vi "Close serial reference.vi"(8 "error in (no error)":errorcluster, 11 "Serial_comms in":refnum<class "Serial_comms.lvclass">) -> (0 "error out":errorcluster, 3 "Serial_comms out":refnum<class "Serial_comms.lvclass">)   [LabVIEW 2020, in "Serial_comms.lvlib" / "Serial_comms.lvclass"]
uses:
  Serial_comms.lvclass
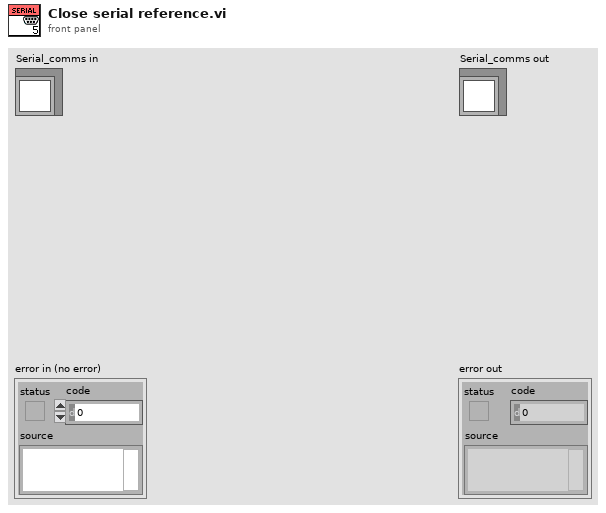
[diagram p1: front panel]
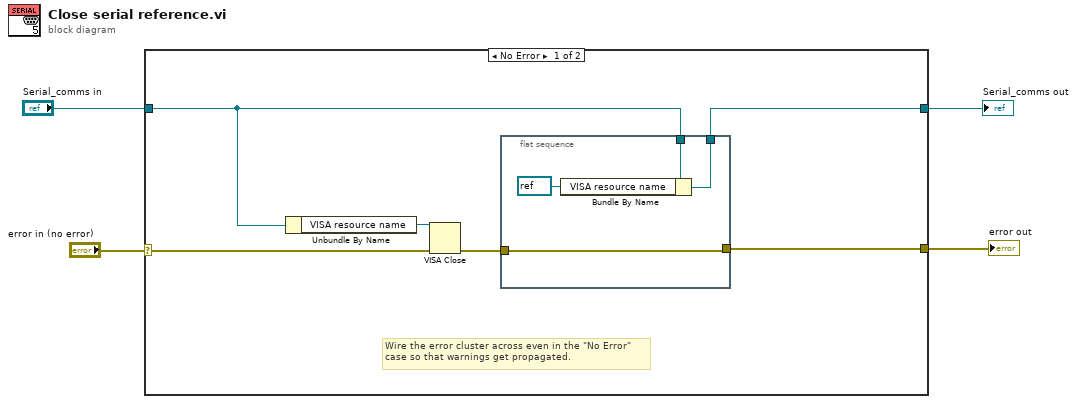
[diagram p0: block diagram]
diagram:
  n1 = case shown="No Error" "error in (no error)" {
    selector: "error in (no error)" -> [w7 w16]
    tunnel: [w6 w16] -> w3
    tunnel: [w5 w15] -> w1
    tunnel: "Serial_comms in" -> [w8 w15]
    frame No Error {
      # "Wire the error cluster across even in the \"No Error\"\ncase so that warnings get propagated."
      n2 = Unbundle By Name(w8) -> ("VISA resource name"=w10:refnum<visa-resource-name>)
      n3 = VISA Close(VISA resource name=w10, error in (no error)=w7) -> (error out=w9:errorcluster)
      n4 = flat-sequence {
        tunnel: w8 -> [w14]
        tunnel: [w12] -> w5
        tunnel: [w11] -> w6
        tunnel: w9 -> [w11]
        frame #0 {
          n5 = Bundle By Name(cluster=w14, "VISA resource name"=refnum<visa-resource-name> refnum) -> (w12:refnum<class "Serial_comms.lvclass">)
        }
      }
    }
    frame Error {
    }
  }
  "error out" <- w3
  "Serial_comms out" <- w1
